vi "LMPop.vi"(0 "reference in":refnum<class "Redis.lvclass">, 1 "Keys":string[](array[string]), 5 "WhereFrom":T1, 9 "Count(1)":u32=1, 11 "Error In":errorcluster) -> (4 "reference out":refnum<class "Redis.lvclass">, 8 "Elements":string[](array[string]), 15 "Error Out":errorcluster)   [LabVIEW 2020, in "Redis.lvclass"]
doc: "<b>LMPOP</b>\n\nPops one or more elements from the first non-empty list key from the list of provided key names.\n\nLMPOP and BLMPOP are similar to the following, more limited, commands:\n\nLPOP or RPOP which take only one key, and can return multiple elements.\nBLPOP or BRPOP which take multiple keys, but return only one element from just one key.\nSee BLMPOP for the blocking variant of this command.\n\nElements are popped from either the left or right of the first non-empty list based on the passed argument. The number of returned elements is limited to the lower between the non-empty list's length, and the <b>count</b> argument (which defaults to 1)."
uses:
  Redis.lvclass
  SideEnum.ctl
  Redis.lvclass/Redis.ctl
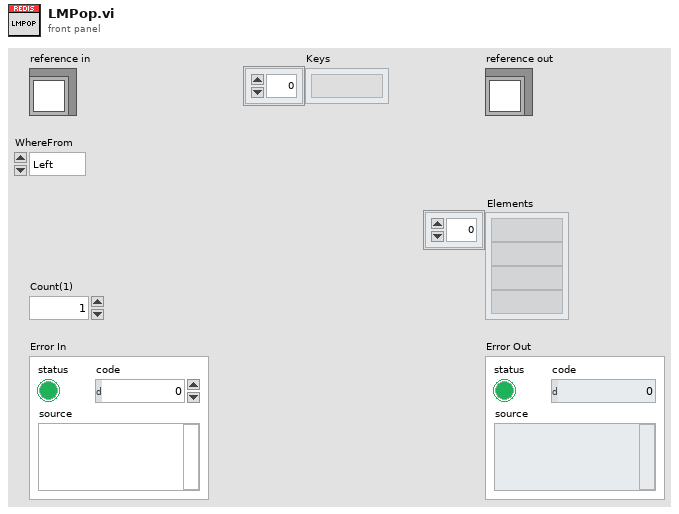
[diagram p1: front panel]
types:
  T1 = typedef "Redis.lvclass/SideEnum.ctl" = enum16{"Left", "Right"}
  T2 = typedef "Redis.lvclass/RedisDataType.ctl" = cluster{"Reply Type":T3, "Integer":i64, "String":string, "Multibulk":variant[], "StringData":string[]}
  T3 = typedef "Redis.lvclass/ReplyDataTypeEnum.ctl" = enum16{"None", "Error", "Status", "Nil", "Integer", "String", "Multibulk"}
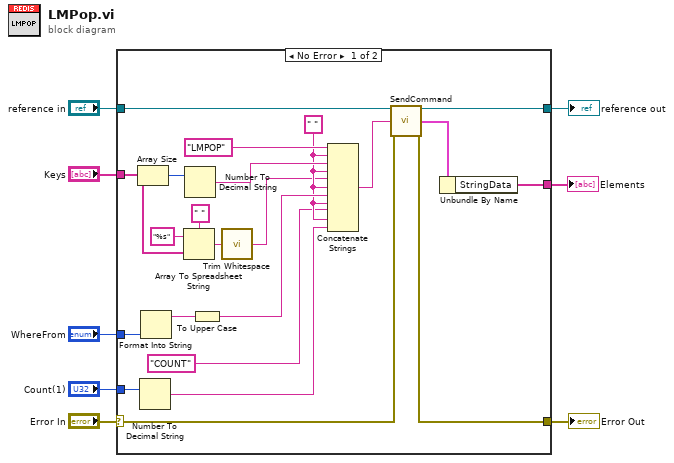
[diagram p0: block diagram]
diagram:
  n1 = case shown="No Error" "Error In" {
    selector: "Error In" -> [w28 w32]
    tunnel: [w27 w32] -> w7
    tunnel: [w30 w31] -> w5
    tunnel: "reference in" -> [w29 w31]
    tunnel: "Keys" -> [w16 _]
    tunnel: [w23 _] -> w3
    tunnel: "Count(1)" -> [w22 _]
    tunnel: "WhereFrom" -> [w18 _]
    frame No Error {
      w12 = " "
      n2 = Array Size(array=w16) -> (size(s)=w21:i32)
      n3 = Number To Decimal String(number=w22) -> (decimal integer string=w10:string)  [unwired: 1 in]
      n4 = Format Into String(w18) -> (resulting string=w19:string)  [unwired: 3 in, 1 out]
      n5 = Array To Spreadsheet String(delimiter (Tab)=" ", array=w16, 3:"%s" ("format string")) -> (spreadsheet string=w14:string)
      n6 = Number To Decimal String(number=w21) -> (decimal integer string=w20:string)  [unwired: 1 in]
      n7 = To Upper Case(1:w19) -> (0:w13:string)
      n8 = call <vilib>:"Trim Whitespace.vi"("string"=w14) -> ("trimmed string"=w9:string)  [unwired: 1 in]
      n9 = Concatenate Strings("LMPOP", w12, w20, w12, w9, w12, w13, w12, "COUNT", w12, w10) -> (w25:string)
      n10 = call "SendCommand.vi"("reference in"=w29, "Command"=w25, "Error In"=w28) -> ("reference out"=w30:refnum<class "Redis.lvclass">, "Data"=w24:T2, "Error Out"=w27:errorcluster)  [unwired: 10 in]
      n11 = Unbundle By Name(w24) -> ("StringData"=w23:string[])
    }
    frame Error {
    }
  }
  "Error Out" <- w7
  "reference out" <- w5
  "Elements" <- w3
